vi "4Pi 4Pi Modes - Get Image Full.vi"(0 "Camera Notifier Name":string, 7 "Image Ref":T1, 11 "Image Dst":T1, 13 "Frame Accums.":u16) -> (8 "Image Dst Out":T1)   [LabVIEW 2016]
uses:
  <vilib>/vision/Image Controls.llb/IMAQ Image.ctl
  Device Library/Cameras/Camera Controls/Generic Camera Actions.ctl
  Device Library/Cameras/Camera Controls/Camera IMAQ Key Info.ctl
  <vilib>/vision/NI_Vision_Development_Module.lvlib
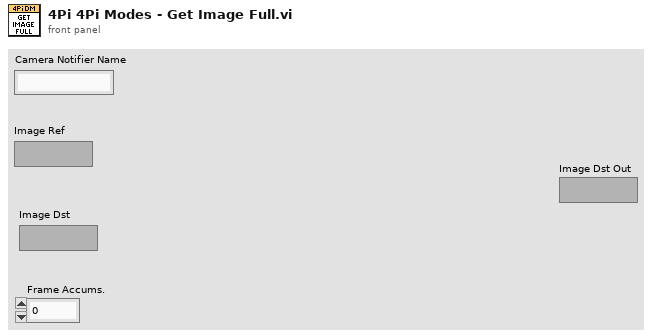
[diagram p1: front panel]
types:
  T1 = typedef "IMAQ Image.ctl" = refnum<image>
  T2 = typedef "Generic Camera Actions.ctl" = enum16{"Status", "Live Preview", "Capture", "Abort", "Set Exposure Time (s)", "Get Exposure Time (s)", "Record Settings", "Set ROI", "Get ROI", "Defect Correction On/Off", "Cooler On/Off", "Fan On/Off", "Quti"}
  T3 = typedef "Camera IMAQ Key Info.ctl" = cluster{"Frame":u32, "Sensor Height":i32, "Sensor Width":i32, "ROI Height":i32, "ROI Width":i32, "ROI Enable?":bool, "Bit per Pixel":u8}
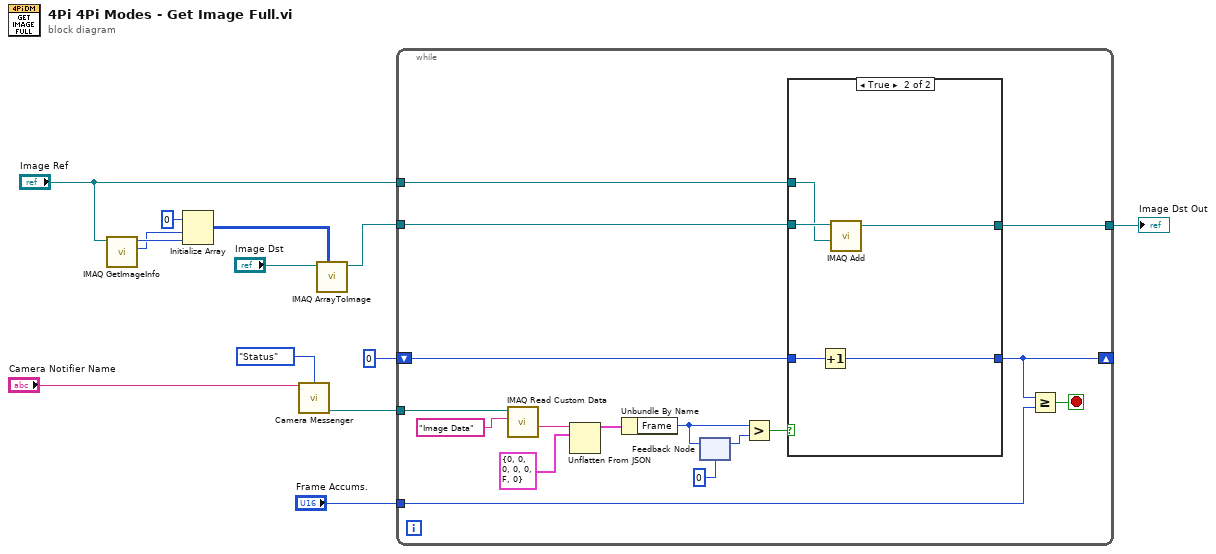
[diagram p0: block diagram]
diagram:
  n1 = call "IMAQ GetImageInfo"("Image"="Image Ref") -> ("Y Resolution"=w6:i32, "X Resolution"=w7:i32)  [unwired: 3 in, 6 out]
  n2 = Initialize Array(u16 0 ("element"), w6, w7) -> (w3:u16[][])
  n3 = call "Camera Messenger.vi"("Notifier Name"="Camera Notifier Name", "General Camera Actions"=Generic_Camera_Actions."Status") -> ("Image Ref"=w12:T1)  [unwired: 8 in, 5 out]
  n4 = call "IMAQ ArrayToImage"("Image Pixels (U16)"=w3, "Image"="Image Dst") -> ("Image Out"=w2:T1)  [unwired: 8 in, 1 out]
  n5 = while {
    tunnel: w12 -> [w25]
    shift-right: [w19] -> _
    shift-left: u16 0 -> [w20]
    tunnel: "Image Ref" -> [w17]
    tunnel: "Frame Accums." -> [w16]
    tunnel: w2 -> [w15]
    tunnel: [w14] -> w9
    stop <- w18 stop-if-true
    n6 = call "IMAQ Read Custom Data"("Key"="Image Data", "Image"=w25) -> ("Custom Data Out"=w27:string)  [unwired: 7 in, 2 out]
    n7 = Unflatten From JSON(JSON string=w27, type and defaults=T3 {"Frame"=0, "Sensor Height"=0, "Sensor Width"=0, "ROI Height"=0, "ROI Width"=0, "ROI Enable?"=FALSE, "Bit per Pixel"=0} ("Camera IMAQ Key Info")) -> (value=w29:T3)  [unwired: 5 in, 1 out]
    n8 = Unbundle By Name(w29) -> ("Frame"=w22:u32)
    n9 = feedback #1(u32 0 ("Frame")) -> (w24:u32)
    n10 = feedback-in #1(w22) -> ()
    n11 = Greater?(x=w22, y=w24) -> (0:w21:bool)
    n12 = case shown="True" w21 {
      tunnel: w20 -> [w31 w36]
      tunnel: [w31 w35] -> w19
      tunnel: w17 -> [_ w33]
      tunnel: w15 -> [w30 w34]
      tunnel: [w30 w32] -> w14
      frame False {
      }
      frame True {
        n13 = Increment(x=w36) -> (x+1=w35:u16)
        n14 = call "IMAQ Add"("Image Src A"=w34, "Image Src B"=w33) -> ("Image Dst Out"=w32:T1)  [unwired: 5 in, 1 out]
      }
    }
    n15 = Greater Or Equal?(x=w19, y=w16) -> (x >= y?=w18:bool)
  }
  "Image Dst Out" <- w9
